vi "DB Tools Update Data.vi"(5 "condition":string, 6 "flatten cluster? (F)":bool, 7 "data":variant, 8 "error in (no error)":errorcluster, 9 "columns":string[](array[string]), 10 "table":string, 11 "connection reference":T1) -> (0 "error out":errorcluster, 3 "connection reference out":T1)   [LabVIEW 2017, in "NI_Database_API.lvlib"]
doc: "Updates the data in a database identified by <B>connection reference</B>."
uses:
  <vilib>/addons/database/NI_Database_API.lvlib
  <vilib>/addons/database/Connection.llb/Conn ObjectReference.ctl
  <vilib>/addons/database/Command.llb/Cmd Execute.vi
  <vilib>/addons/database/Recordset.llb/Rec Destroy - Command.vi
  <vilib>/addons/database/Command.llb/Cmd Delete.vi
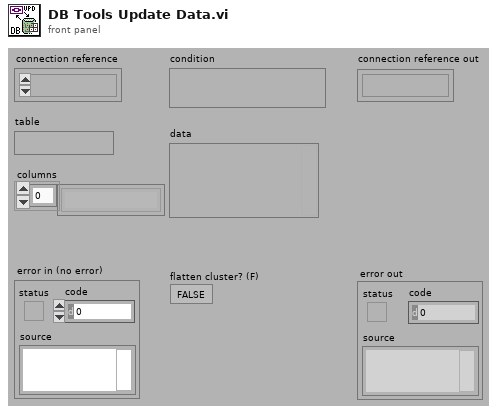
[diagram p1: front panel]
types:
  T1 = typedef "NI_Database_API.lvlib/Conn ObjectReference.ctl" = refnum<k1>
  T2 = typedef "NI_Database_API.lvlib/DB Tools Parameter Info.ctl" = cluster{"parameter name":string, "type":T3, "direction":T4, "value":variant}
  T3 = typedef "NI_Database_API.lvlib/DB Tools DataTypes.ctl" = enum16{"String", "Long (I32)", "Single (SGL)", "Double (DBL)", "Date/Time", "Binary"}
  T4 = typedef "NI_Database_API.lvlib/DB Tools Parameter Dir.ctl" = enum32{"Input", "Output", "Input/Output", "Return Value"}
  T5 = typedef "NI_Database_API.lvlib/Cmd ObjectReference.ctl" = refnum<k1>
  T6 = typedef "NI_Database_API.lvlib/Cmd-Rec Object Reference.ctl" = refnum<k1>
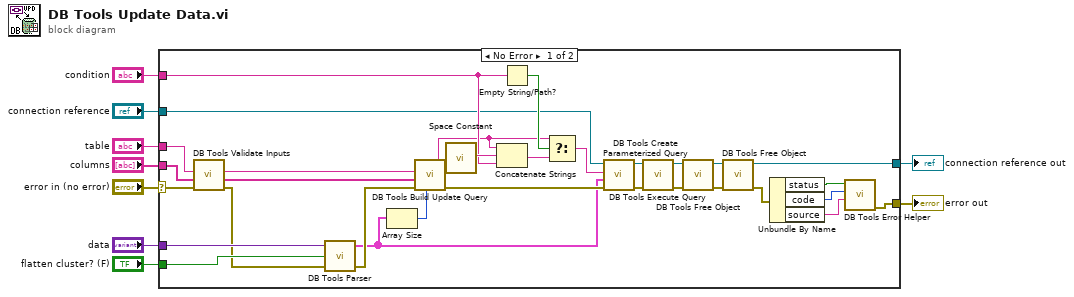
[diagram p0: block diagram]
diagram:
  n1 = case shown="No Error" "error in (no error)" {
    selector: "error in (no error)" -> [w13 w42]
    tunnel: "table" -> [w40 _]
    tunnel: [w39 w41] -> w8
    tunnel: "data" -> [w38 _]
    tunnel: "flatten cluster? (F)" -> [w37 _]
    tunnel: "connection reference" -> [w12 w41]
    tunnel: "columns" -> [w26 _]
    tunnel: [w22 w42] -> w3
    tunnel: "condition" -> [w17 _]
    frame No Error {
      n2 = call <vilib>:"DB Tools Validate Inputs.vi"("error in (no error)"=w13, "columns"=w26, "table"=w40) -> ("error out"=w10:errorcluster, "columns out"=w11:string[], "table out"=w27:string)  [unwired: 2 in]
      n3 = call <vilib>:"DB Tools Parser.vi"("error in (no error)"=w10, "flatten cluster? (F)"=w37, "variant"=w38) -> ("error out"=w28:errorcluster, "parameters"=w15:T2[])  [unwired: 1 in]
      n4 = Array Size(array=w15) -> (size(s)=w29:i32)
      n5 = call <vilib>:"DB Tools Build Update Query.vi"("num parameters"=w29, "error in (no error)"=w28, "columns"=w11, "table name"=w27) -> ("error out"=w30:errorcluster, "query"=w16:string)  [unwired: 3 in]
      n6 = call <vilib>:"Space Constant.vi"() -> ("String"=w19:string)
      n7 = Concatenate Strings(w16, w19, w17) -> (w20:string)
      n8 = Empty String/Path?(string/path=w17) -> (empty?=w21:bool)
      n9 = Select(t=w16, s=w21, f=w20) -> (s? t:f=w18:string)
      n10 = call <vilib>:"DB Tools Create Parameterized Query.vi"("error in (no error)"=w30, "parameters"=w15, "SQL query"=w18, "connection reference"=w12) -> ("error out"=w35:errorcluster, "command reference"=w34:T5)  [unwired: 3 in, 1 out]
      n11 = call-poly <vilib>:"DB Tools Execute Query.vi"("error in (no error)"=w35, "command reference"=w34) -> ("error out"=w32:errorcluster, "command-recordset reference"=w33:T6)  [unwired: 6 in]
      n12 = call-poly <vilib>:"DB Tools Free Object.vi"("error in (no error)"=w32, "command-recordset reference"=w33) -> ("error out"=w36:errorcluster, "command reference"=w31:T5)  [unwired: 8 in]
      n13 = call-poly <vilib>:"DB Tools Free Object.vi"("error in (no error)"=w36, "command reference"=w31) -> ("error out"=w23:errorcluster, "connection reference"=w39:T1)  [unwired: 8 in]
      n14 = Unbundle By Name(w23) -> ("status"=w25:bool, "code"=w14:i32, "source"=w24:string)
      n15 = call <vilib>:"DB Tools Error Helper.vi"("source"=w24, "code"=w14, "status"=w25) -> ("error out"=w22:errorcluster)  [unwired: 8 in]
    }
    frame Error {
    }
  }
  "error out" <- w3
  "connection reference out" <- w8
